vi "Get Status.vi"(8 "error in (no error)":errorcluster, 11 "Instrument.1820 in":refnum<class "Instrument.OxfordVRM.lvclass">) -> (0 "error out":errorcluster, 1 "Status":T1, 2 "Status":string, 3 "Instrument.1820 in":refnum<class "Instrument.OxfordVRM.lvclass">)   [LabVIEW 2016, in "Instrument.OxfordVRM.lvclass"]
doc: "Status Bits:\n[0] = Hold?\n[1] = Ramp to Set?\n[2] = Ramp to Zero?\n[3] = Clamp?"
uses:
  Instrument.OxfordVRM.lvclass
  Typedefs/Instrument.Oxford1820.Commands-enum.ctl
  <instrlib>/Mercury iXX/Public/Libraries/Magnet/Controls/PSU Actions.ctl
  <instrlib>/Mercury iXX/Public/Libraries/Magnet.lvlib
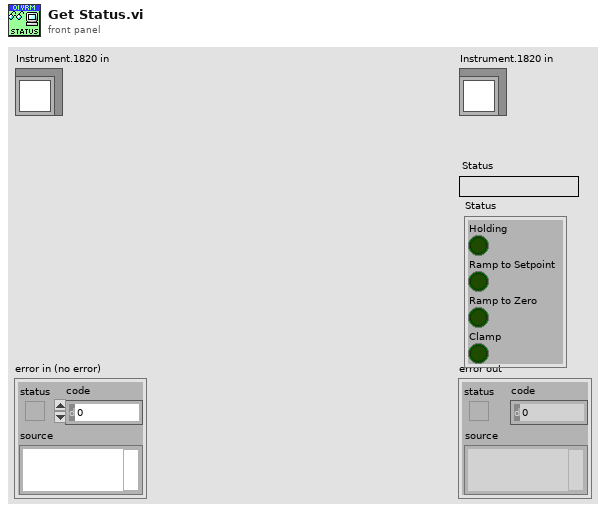
[diagram p1: front panel]
types:
  T1 = cluster{"Holding":bool, "Ramp to Setpoint":bool, "Ramp to Zero":bool, "Clamp":bool}
  T2 = typedef "Instrument.OxfordVRM.lvclass/Instrument.Oxford1820.Commands-enum.ctl" = enum16{"setAction", "setTarget", "setSwitchHeat", "setLambda", "setFillMode", "setNeedleValve", "setMagnetField", "getStatus", "getTarget", "getSwitchHeat", "getPSUField", "newcommand", "getMagnetField"}
  T3 = typedef "Mercury iXX.lvlib/Magnet.lvlib/PSU Actions.ctl" = string
  T4 = cluster{"[0]":bool, "[1]":bool, "[2]":bool, "[3]":bool}
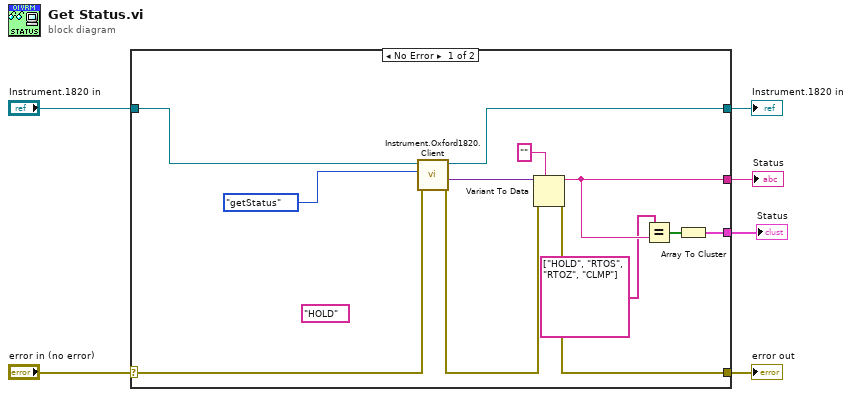
[diagram p0: block diagram]
diagram:
  n1 = case shown="No Error" "error in (no error)" {
    selector: "error in (no error)" -> [w17 w20]
    tunnel: [w14 w20] -> w5
    tunnel: [w7 w19] -> w3
    tunnel: "Instrument.1820 in" -> [w8 w19]
    tunnel: [w12 _] -> w2
    tunnel: [w9 _] -> w1
    frame No Error {
      (unwired) T3 "HOLD" ("PSU Act Stat")
      n2 = call "Instrument.Oxford1820.Client.vi"("error in (no error)"=w17, "Commands"=Instrument.Oxford1820.Commands-enum."getStatus", "Instrument.1820 in"=w8) -> ("error out"=w15:errorcluster, "Data out"=w16:variant, "Instrument.1820 out"=w7:refnum<class "Instrument.OxfordVRM.lvclass">)  [unwired: 6 in]
      n3 = Variant To Data(error in=w15, type="", Variant=w16) -> (data=w12:string, error out=w14:errorcluster)
      n4 = Equal?(x=string[] ["HOLD", "RTOS", "RTOZ", "CLMP"] ("Array"), y=w12) -> (x = y?=w10:bool[])
      n5 = Array To Cluster(array=w10) -> (cluster=w9:T4)
    }
    frame Error {
    }
  }
  "error out" <- w5
  "Instrument.1820 in" <- w3
  "Status" <- w2
  "Status" <- w1
